vi "COM write file.vi"(10 "COM file path":path, 11 "COM Port:":refnum<visa-resource-name>="COM3") -> ()   [LabVIEW 2020]
panel:
  out "COM port string":string
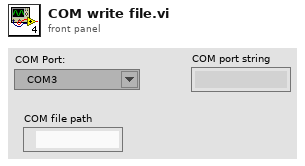
[diagram p1: front panel]
types:
  T1 = enum16{"open", "replace", "create", "open or create", "replace or create", "replace or create with confirmation"}
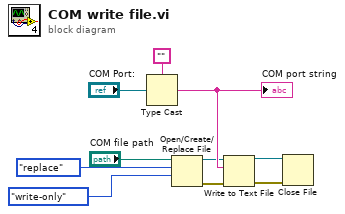
[diagram p0: block diagram]
diagram:
  n1 = Type Cast(type="", x="COM Port:") -> (*(type *) &x=w7:string)
  "COM port string" <- w7
  n2 = Open/Create/Replace File(file path (use dialog)="COM file path", operation (0:open)=T1."replace", access (0:read/write)=enum16{"read/write", "read-only", "write-only"}."write-only") -> (refnum out=w6:refnum<file>, error out=w5:errorcluster)  [unwired: 3 in, 1 out]
  n3 = Write to Text File(file (use dialog)=w6, text=w7, error in=w5) -> (refnum out=w4:refnum<file>, error out=w3:errorcluster)  [unwired: 1 in, 1 out]
  n4 = Close File(refnum=w4, error in=w3) -> ()  [unwired: 2 out]
